vi "Populate Attribute Details.vi"(8 "error in":errorcluster, 9 "Sub-Index":string, 10 "Index":string, 11 "UI Actor in":refnum<class "UI Actor.lvclass">) -> (0 "error out":errorcluster, 3 "UI Actor out":refnum<class "UI Actor.lvclass">)   [LabVIEW 2024, in "UI Actor.lvlib" / "UI Actor.lvclass"]
uses:
  UI Actor.lvclass
  UI Actor.lvclass/UI Actor.ctl
  Core/EDS/EDS.lvclass
  Core/Sorted Object Dictionary/Sorted Object Dictionary.lvclass
  Core/OD Entry/OD Entry.lvclass
  Core/OD Sub-Entry/OD Sub-Entry.lvclass
  D:/git/EDS-File-Viewer/Core/OD Entry/OD Entry.lvclass
  D:/git/EDS-File-Viewer/Core/OD Sub-Entry/OD Sub-Entry.lvclass
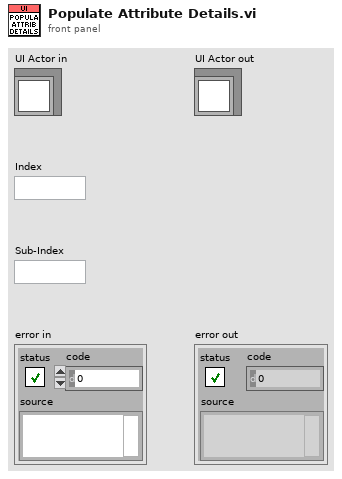
[diagram p1: front panel]
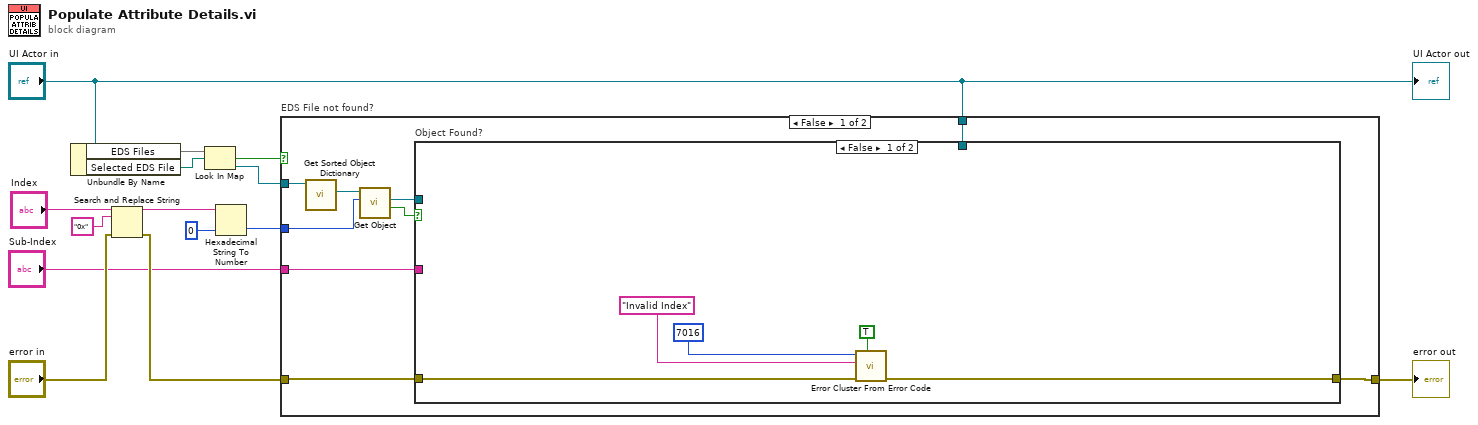
[diagram p0: block diagram]
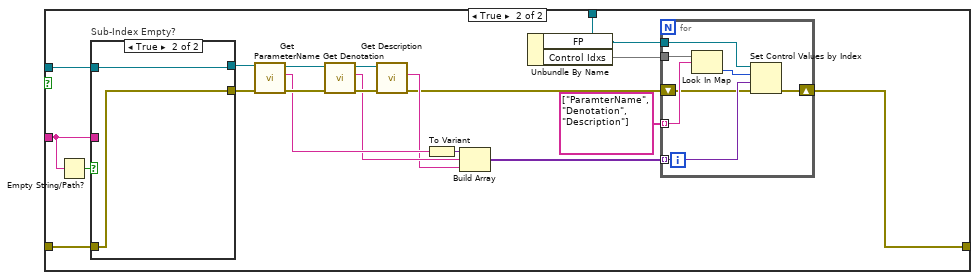
[diagram p2: hidden frame]
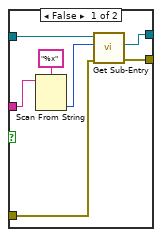
[diagram p3: hidden frame]
diagram:
  n1 = Unbundle By Name("UI Actor in") -> ("EDS Files"=w14:map{path, refnum<class "EDS.lvclass">}, "Selected EDS File"=w13:path)
  n2 = Search and Replace String(input string="Index", search string="0x", error in="error in") -> (result string=w4:string, error out=w6:errorcluster)  [unwired: 5 in, 2 out]
  n3 = Look In Map(map=w14, key=w13) -> (key not found?=w5:bool, value=w12:refnum<class "EDS.lvclass">)  [unwired: 1 in]
  n4 = Hexadecimal String To Number(string=w4, default (0uL)=u16 0) -> (number=w3:u16)  [unwired: 1 in, 1 out]
  n5 = case "EDS File not found?" shown="False" w5 {
    tunnel: w12 -> [w23 _]
    tunnel: w6 -> [w22 w66]
    tunnel: [w15 w66] -> w10
    tunnel: "UI Actor in" -> [w16 _]
    tunnel: w3 -> [w21 _]
    tunnel: "Sub-Index" -> [w17 _]
    frame False {
      n6 = call "Get Sorted Object Dictionary.vi"("EDS in"=w23) -> ("Sorted Object Dictionary"=w18:refnum<class "Sorted Object Dictionary.lvclass">)  [unwired: 9 in, 1 out]
      n7 = call "Get Object.vi"("Numeric"=w21, "Sorted Object Dictionary in"=w18) -> ("Found?"=w19:bool, "OD Entry"=w20:refnum<class "OD Entry.lvclass">)  [unwired: 7 in, 1 out]
      n8 = case "Object Found?" shown="False" w19 {
        tunnel: w22 -> [w28 w48]
        tunnel: w20 -> [_ w49]
        tunnel: w17 -> [_ w46]
        tunnel: w16 -> [_ w42]
        tunnel: [w24 w29] -> w15
        frame False {
          n9 = call <vilib>:"Error Cluster From Error Code.vi"("show call chain? (False)"=TRUE, "error in (no error)"=w28, "error message (\"\")"="Invalid Index" ("error message (\"\")"), "error code (0)"=7016) -> ("error out"=w24:errorcluster)  [unwired: 5 in]
        }
        frame True {
          n10 = Empty String/Path?(string/path=w46) -> (empty?=w47:bool)
          n11 = case "Sub-Index Empty?" shown="True" w47 {
            tunnel: w49 -> [w63 w65]
            tunnel: w48 -> [w59 w64]
            tunnel: w46 -> [w60 _]
            tunnel: [w58 w65] -> w40
            tunnel: [w57 w64] -> w43
            frame False {
              n12 = Scan From String(format string="%x", input string=w60) -> (output 1=w61:u16)  [unwired: 3 in, 3 out]
              n13 = call "Get Sub-Entry.vi"("Error In"=w59, "Sub-Index"=w61, "reference in"=w63) -> ("Error Out"=w57:errorcluster, "OD Sub-Entry"=w58:refnum<class "OD Sub-Entry.lvclass">)  [unwired: 5 in, 2 out]
            }
            frame True {
            }
          }
          n14 = call "Get ParameterName.vi"("Error In"=w43, "reference in"=w40) -> ("Error Out"=w41:errorcluster, "ParameterName"=w37:string, "reference out"=w39:refnum<class "OD Entry.lvclass">)  [unwired: 6 in, 1 out]
          n15 = call "Get Denotation.vi"("Error In"=w41, "reference in"=w39) -> ("Error Out"=w45:errorcluster, "Denotation"=w36:string, "reference out"=w44:refnum<class "OD Entry.lvclass">)  [unwired: 7 in]
          n16 = call "Get Description.vi"("Error In"=w45, "reference in"=w44) -> ("Error Out"=w30:errorcluster, "Description"=w35:string)  [unwired: 7 in, 1 out]
          n17 = To Variant(anything=w37) -> (Variant=w33:variant)
          n18 = Build Array(w33, w36, w35) -> (w34:variant[])
          n19 = Unbundle By Name(w42) -> ("FP"=w31:refnum<vi>, "Control Idxs"=w38:map{string, i32})
          n20 = for {
            tunnel: w38 -> [w56]
            tunnel: w34 -> [w54] mode=indexing
            tunnel: string[] ["ParamterName", "Denotation", "Description"] -> [w53] mode=indexing
            tunnel: w31 -> [w52]
            shift-right: [w50] -> w29
            shift-left: w30 -> [w51]
            n21 = Look In Map(map=w56, key=w53) -> (value=w55:i32)  [unwired: 1 in, 1 out]
            n22 = Set Control Values by Index(0:w52, 1:w55, 2:w54, 3:w51) -> (11:w50:errorcluster)
          }
        }
      }
    }
    frame True {
    }
  }
  "error out" <- w10
  "UI Actor out" <- "UI Actor in"
